vi "CryoServer Send Command.vi"(8 "error in (no error)":errorcluster, 10 "command string":string, 11 "connection ID":refnum<k5>) -> (0 "error out":errorcluster, 2 "Response":string, 3 "connection ID out":refnum<k5>)   [LabVIEW 2024, in "CryoServer.lvclass"]
uses:
  CryoServer.lvclass
  <vilib>/Utility/error.llb/Trim Whitespace One-Sided.vi
  <vilib>/JDP Science/JSONtext/Next JSON Value.vi
  <vilib>/JDP Science/JSONtext/String Subset.vi
  <vilib>/JDP Science/JSONtext/Parsing/Advance past next JSON Value (inlined COPY).vi
  <vilib>/JDP Science/JSONtext/Parsing/Advance past whitespace.vi
  <vilib>/JDP Science/JSONtext/Parsing/Advance past String.vi
  <vilib>/JDP Science/JSONtext/Parsing/Advance past Number.vi
  <vilib>/JDP Science/JSONtext/Parsing/Advance past Line Ending.vi
  <vilib>/JDP Science/JSONtext/Parsing/Parse Full Path or Item Name.vi
  <vilib>/JDP Science/JSONtext/Parsing/Advance past Array.vi
  <vilib>/JDP Science/JSONtext/Parsing/Advance past Object.vi
  <vilib>/JDP Science/JSONtext/support/Error Cluster From Code.vi
  <vilib>/JDP Science/JSONtext/Offset/Find Item Locations by Path.vi
  <vilib>/JDP Science/JSONtext/JSONtext.lvlib
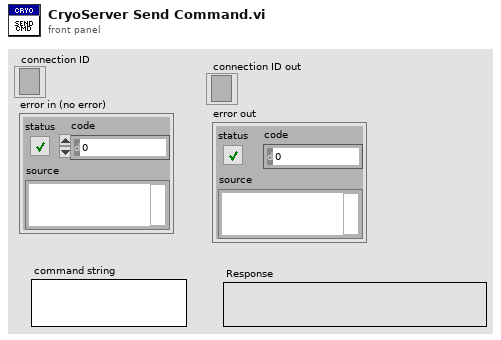
[diagram p1: front panel]
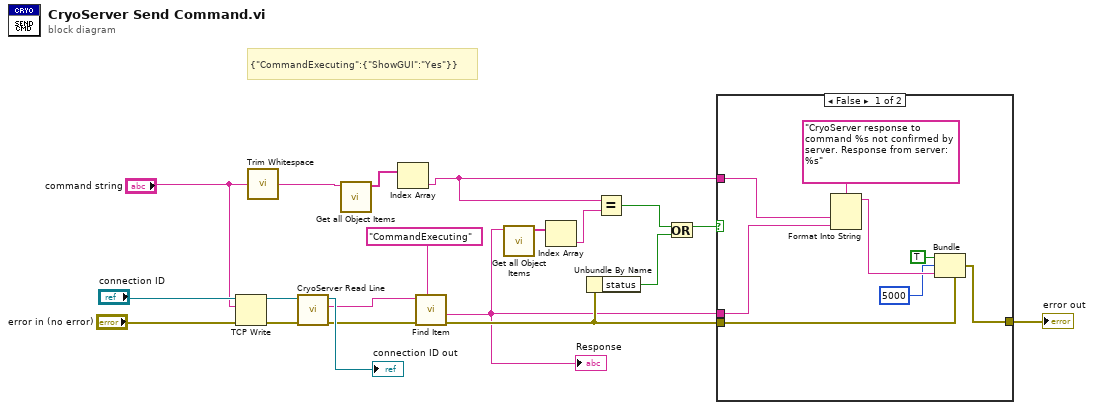
[diagram p0: block diagram]
diagram:
  # "{\"CommandExecuting\":{\"ShowGUI\":\"Yes\"}}"
  n1 = TCP Write(connection ID="connection ID", data in="command string", error in (no error)="error in (no error)") -> (connection ID out=w11:refnum<k5>, error out=w12:errorcluster)  [unwired: 1 in, 1 out]
  n2 = call <vilib>:"Trim Whitespace.vi"("string"="command string") -> ("trimmed string"=w5:string)  [unwired: 1 in]
  n3 = call "CryoServer Read Line.vi"("error in (no error)"=w12, "connection ID"=w11) -> ("error out"=w9:errorcluster, "data out"=w8:string, "connection ID out"=→"connection ID out":refnum<k5>)  [unwired: 7 in]
  n4 = call <vilib>:"Get all Object Items.vi"("JSON"=w5) -> ("Item Names"=w4:string[])  [unwired: 7 in, 3 out]
  n5 = Index Array(array=w4) -> (element=w3:string)  [unwired: 1 in]
  n6 = call <vilib>:"Find Item.vi"("$Path or Item Name"="CommandExecuting", "error in (no error)"=w9, "JSON"=w8) -> ("error out"=w7:errorcluster, "<JSON>"=w6:string)  [unwired: 5 in, 2 out]
  "Response" <- w6
  n7 = call <vilib>:"Get all Object Items.vi"("JSON"=w6) -> ("Item Names"=w2:string[])  [unwired: 7 in, 3 out]
  n8 = Index Array(array=w2) -> (element=w1:string)  [unwired: 1 in]
  n9 = Unbundle By Name(w7) -> ("status"=w15:bool)
  n10 = Equal?(x=w3, y=w1) -> (x = y?=w13:bool)
  n11 = Or(x=w13, y=w15) -> (x .or. y?=w16:bool)
  n12 = case shown="False" w16 {
    tunnel: w7 -> [w25 w29]
    tunnel: [w24 w29] -> w14
    tunnel: w3 -> [w27 _]
    tunnel: w6 -> [w26 _]
    frame False {
      n13 = Format Into String(format string="CryoServer response to command %s not confirmed by server. Response from server: %s", w27, w26) -> (resulting string=w22:string)  [unwired: 2 in, 1 out]
      n14 = Bundle(cluster=w25, "status"=TRUE, "code"=5000, "source"=w22) -> (w24:errorcluster)
    }
    frame True {
    }
  }
  "error out" <- w14
